vi "InterpolateLithographyPoints.vi"(8 "error in (no error)":errorcluster, 11 "Asylum_Driver in":refnum<class "Asylum_Driver.lvclass">) -> (0 "error out":errorcluster, 3 "Asylum_Driver out":refnum<class "Asylum_Driver.lvclass">)   [LabVIEW 2019, in "Asylum_Driver.lvclass"]
uses:
  Asylum_Driver.lvclass
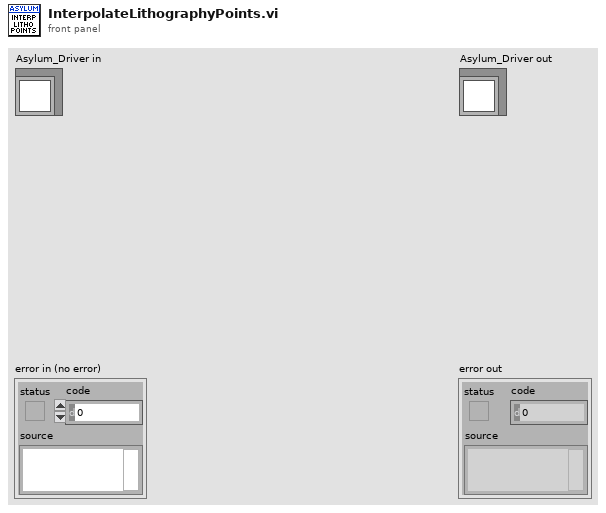
[diagram p1: front panel]
types:
  T1 = typedef "Relay-Box.lvclass/Resistor--enum.ctl" = enum16{"open", "discharge tip", "0 ohms", "100k ohm", "10M ohm", "1G ohm"}
  T2 = cluster{"Name":string, "Litho":cluster{"X":dbl, "Y":dbl, "Speed":dbl, "Voltage":dbl}[], "Set Resistance":T1, "Meta":variant}
  T3 = cluster{"X":dbl, "Y":dbl, "Speed":dbl, "Voltage":dbl}[]
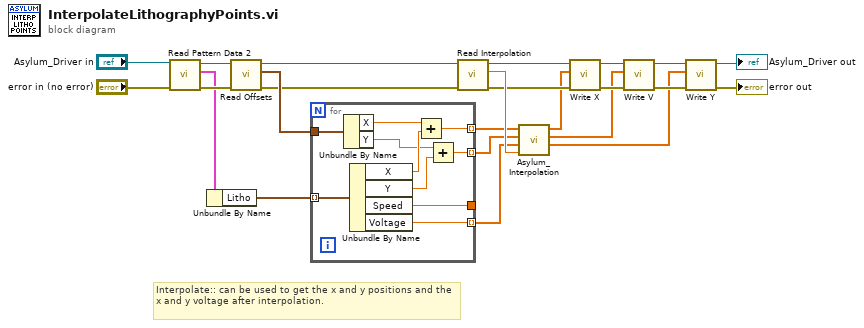
[diagram p0: block diagram]
diagram:
  # "Interpolate:: can be used to get the x and y positions and the x and y voltage after interpolation."
  n1 = call-dynamic "Read Pattern Data 2.vi"("error in (no error)"="error in (no error)", "AFM_Driver in"="Asylum_Driver in") -> ("error out"=w24:errorcluster, "Pattern Data"=w20:T2, "AFM_Driver out"=w23:refnum<class "Asylum_Driver.lvclass">)  [unwired: 7 in]
  n2 = Unbundle By Name(w20) -> ("Litho"=w21:T3)
  n3 = call-dynamic "Read Offsets.vi"("error in (no error)"=w24, "AFM_Driver in"=w23) -> ("error out"=w18:errorcluster, "Offsets"=w22:cluster{"X":dbl, "Y":dbl}, "AFM_Driver out"=w19:refnum<class "Asylum_Driver.lvclass">)  [unwired: 7 in]
  n4 = for {
    tunnel: w21 -> [w34] mode=indexing
    tunnel: [w33] -> _
    tunnel: [w32] -> w16 mode=indexing
    tunnel: w22 -> [w30]
    tunnel: [w26] -> w14 mode=indexing
    tunnel: [w25] -> w15 mode=indexing
    n5 = Unbundle By Name(w30) -> ("X"=w28:dbl, "Y"=w27:dbl)
    n6 = Unbundle By Name(w34) -> ("X"=w31:dbl, "Y"=w29:dbl, "Speed"=w33:dbl, "Voltage"=w32:dbl)
    n7 = Add(x=w28, y=w31) -> (x+y=w26:dbl)
    n8 = Add(x=w27, y=w29) -> (x+y=w25:dbl)
  }
  n9 = call-dynamic "Read Interpolation.vi"("error in (no error)"=w18, "AFM_Driver in"=w19) -> ("error out"=w5:errorcluster, "Interpolation"=w17:dbl, "AFM_Driver out"=w7:refnum<class "Asylum_Driver.lvclass">)  [unwired: 7 in]
  n10 = call "Asylum_Interpolation.vi"("X"=w14, "Y"=w15, "V"=w16, "Interpolation"=w17) -> ("X"=w3:dbl[], "Y"=w2:dbl[], "V"=w1:dbl[])  [unwired: 4 in]
  n11 = call-dynamic "Write X.vi"("error in (no error)"=w5, "X"=w3, "Asylum_Driver in"=w7) -> ("error out"=w10:errorcluster, "Asylum_Driver out"=w11:refnum<class "Asylum_Driver.lvclass">)  [unwired: 7 in]
  n12 = call-dynamic "Write V.vi"("error in (no error)"=w10, "V"=w2, "Asylum_Driver in"=w11) -> ("error out"=w8:errorcluster, "Asylum_Driver out"=w9:refnum<class "Asylum_Driver.lvclass">)  [unwired: 7 in]
  n13 = call-dynamic "Write Y.vi"("error in (no error)"=w8, "Y"=w1, "Asylum_Driver in"=w9) -> ("error out"=→"error out":errorcluster, "Asylum_Driver out"=→"Asylum_Driver out":refnum<class "Asylum_Driver.lvclass">)  [unwired: 7 in]
